vi "Test Write.vi"() -> ()   [LabVIEW 2016]
uses:
  Data/Typedefs/File Type--enum.ctl
  Data/Data.lvclass
panel:
  in  "Append Index":i32
  in  "Notes":string
  in  "path":path
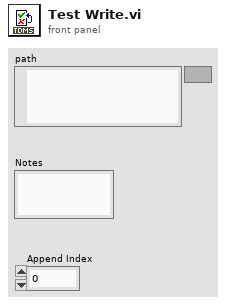
[diagram p1: front panel]
types:
  T1 = typedef "Data.lvclass/File Type--enum.ctl" = enum16{"DAT", "ITX", "TDMS", "VI"}
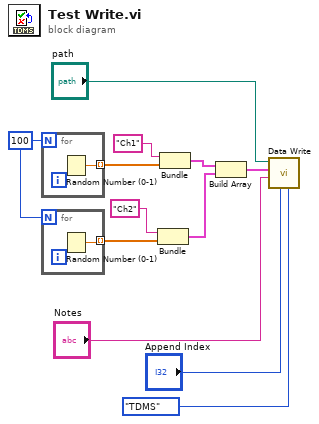
[diagram p0: block diagram]
diagram:
  w8 = 100
  n1 = for {
    N: w8 -> [_]
    tunnel: [w13] -> w6 mode=indexing
    n2 = Random Number (0-1)() -> (number: 0 to 1=w13:dbl)
  }
  n3 = for {
    N: w8 -> [_]
    tunnel: [w14] -> w5 mode=indexing
    n4 = Random Number (0-1)() -> (number: 0 to 1=w14:dbl)
  }
  n5 = Bundle("Ch2", w5) -> (w2:cluster{string, dbl[]})  [unwired: 1 in]
  n6 = Bundle("Ch1", w6) -> (w3:cluster{string, dbl[]})  [unwired: 1 in]
  n7 = Build Array(w3, w2) -> (w4:cluster{string, dbl[]}[])
  n8 = call "Data Write.vi"("File Type"=File_Type--enum."TDMS", "Append Index"="Append Index", "Notes"="Notes", "Data (Dictionary)"=w4, "path"="path") -> ()  [unwired: 5 in, 2 out]
